vi "Read and Calc Analog.vi"() -> ()   [LabVIEW 2013]
panel:
  in  "Знаков после запятой":i32
  out "Результат измерений, В":string
  out "Относительная погрешность, %":dbl
  out "Абсолютная погрешность, В":dbl
  in  "Класс точности (привед. погр.)":dbl
  out "Диапазон измерений, В":dbl
  out "Показания вольтметра, В":dbl
  out "Шкала вольтметра":dbl(knob) scale=0.0..150.0
  in  "Выбор предела измерений":i32(knob)=8 min=0 max=8 step=1 scale=0.0..8.0
  in  "Вариант":T1(ring)
  # "Обработка показаний аналогового вольтметра"
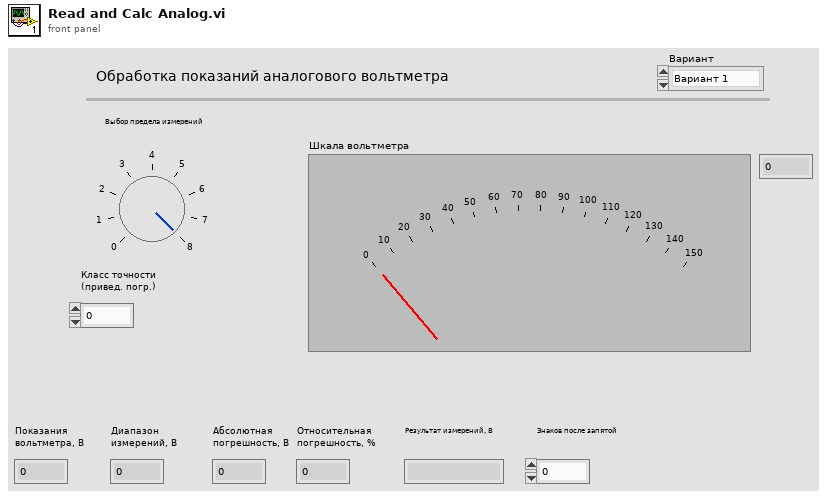
[diagram p1: front panel]
types:
  T1 = enum16{"Вариант 1", "Вариант 2", "Вариант 3", "Вариант 4", "Вариант 5", "Вариант 6", "Вариант 7", "Вариант 8", "Вариант 9", "Вариант 10", "Вариант 11", "Вариант 12"}
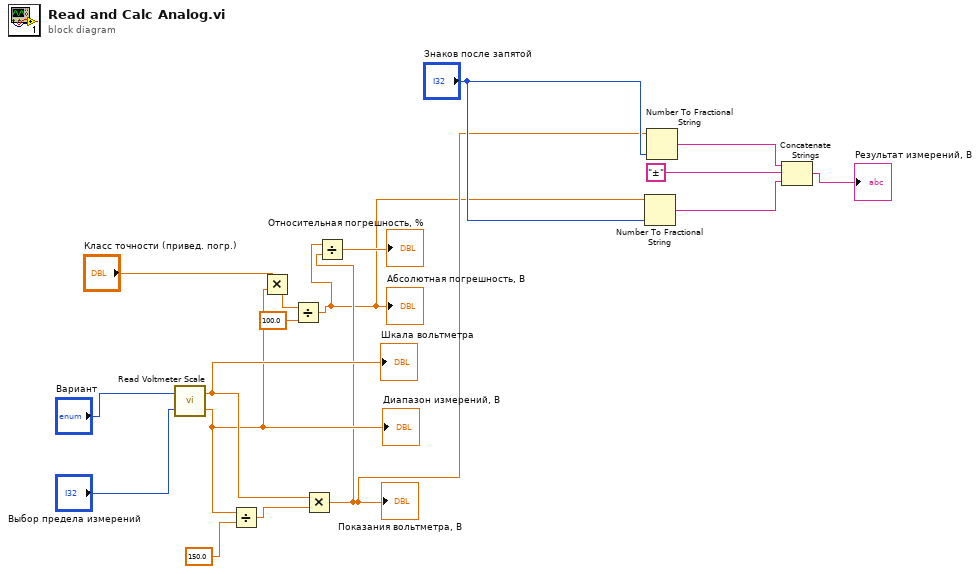
[diagram p0: block diagram]
diagram:
  n1 = call "Read Voltmeter Scale.vi"("Предел"="Выбор предела измерений", "Вариант"="Вариант") -> ("Установленный предел"=w11:dbl, "Положение указателя"=w13:dbl)
  "Шкала вольтметра" <- w13
  "Диапазон измерений, В" <- w11
  n2 = Divide(x=w11, y=150.0) -> (x/y=w14:dbl)
  n3 = Multiply(x="Класс точности (привед. погр.)", y=w11) -> (x*y=w8:dbl)
  n4 = Divide(x=w8, y=100.0) -> (x/y=w5:dbl)
  "Абсолютная погрешность, В" <- w5
  n5 = Multiply(x=w13, y=w14) -> (x*y=w6:dbl)
  "Показания вольтметра, В" <- w6
  n6 = Divide(x=w5, y=w6) -> (x/y=→"Относительная погрешность, %":dbl)
  n7 = Number To Fractional String(number=w5, precision (6)="Знаков после запятой") -> (F-format string=w2:string)  [unwired: 2 in]
  n8 = Number To Fractional String(number=w6, precision (6)="Знаков после запятой") -> (F-format string=w4:string)  [unwired: 2 in]
  n9 = Concatenate Strings(w4, "±", w2) -> (→"Результат измерений, В":string)
